vi "MainExpTrainCode.vi"() -> ()   [LabVIEW 2013]
uses:
  <vilib>/Utility/error.llb/DialogType.ctl
  <vilib>/DAQmx/write.llb/DAQmx Write (Analog Wfm 1Chan NSamp).vi
  <vilib>/DAQmx/create/channels.llb/DAQmx Create Channel (AO-Voltage-Basic).vi
  <vilib>/DAQmx/configure/timing.llb/DAQmx Timing (Sample Clock).vi
  <vilib>/DAQmx/miscellaneous.llb/DAQmx Fill In Error Info.vi
  <resource>/objmgr/daqmx.rc
  <vilib>/measure/NI_MAPro.lvlib
panel:
  in  "offset (volt)":dbl format="%0.2p"
  in  "Time Constant (us)":dbl=50.0
  in  "frequency (Hz)":dbl=10.0 format="%0.2p"
  in  "amplitude (volt)":dbl=1.0 format="%0.2p"
  in  "Number of Samples":i32=1000
  in  "Clock Source":tag="OnboardClock"
  out "Actual Sampling rate (S/s)":dbl=200000.0
  in  "Sample rate( S/s)":dbl=200000.0 format="%0.2f"
  out "Waveform Chart":waveform(dbl)(graph)={"t0"=timestamp(0 s since 1904-01-01), "dt"=5e-06, "Y"=array[1000 elements]}
  in  "stop":bool
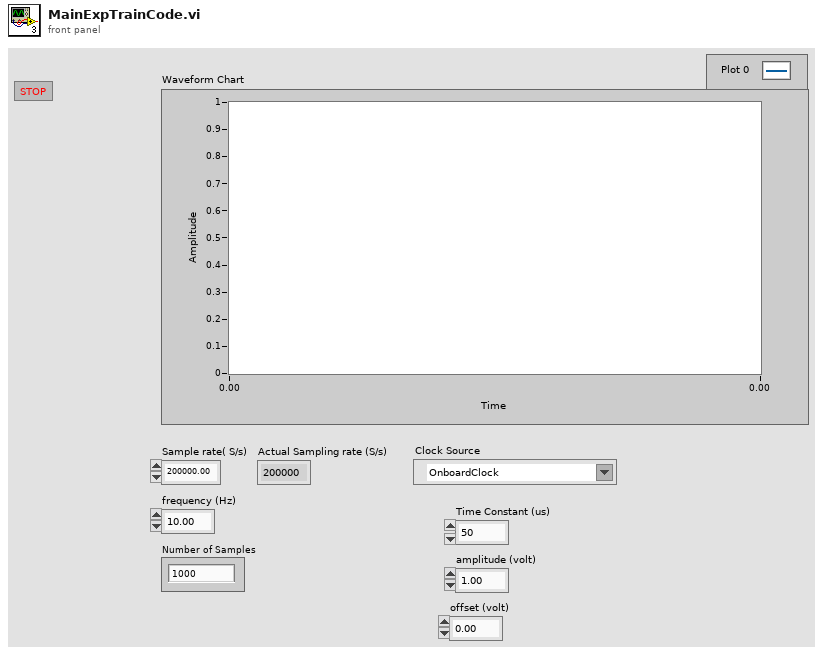
[diagram p1: front panel]
types:
  T1 = typedef "DialogType.ctl" = u16
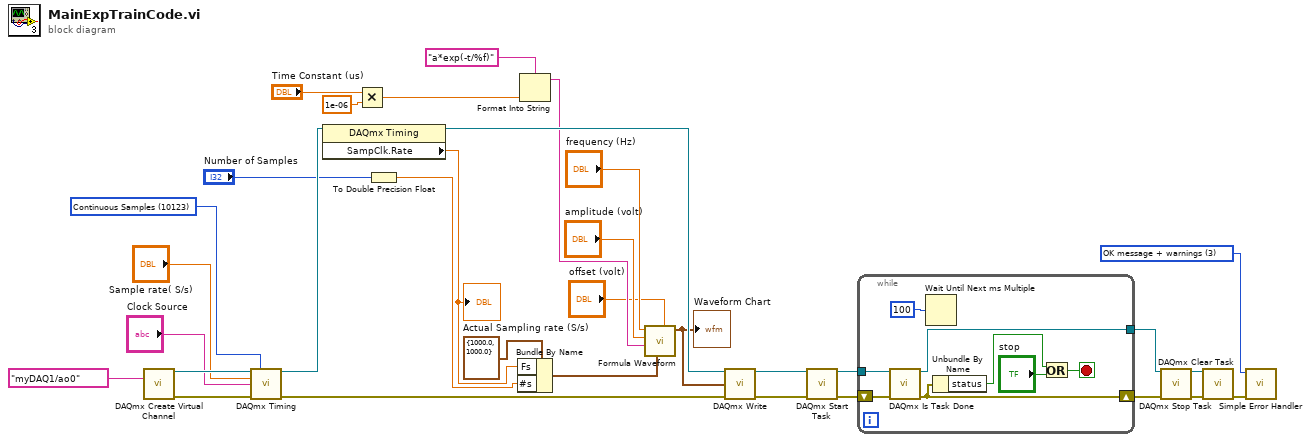
[diagram p0: block diagram]
diagram:
  w10 = T1 3 items=["no dialog", "OK message", "continue or stop message", "OK message + warnings", "continue/stop + warnings"] ("type of dialog (OK msg:1)")
  w32 = 10123 items=["Finite Samples"=10178, "Continuous Samples"=10123, "Hardware Timed Single Point"=12522] ("sample mode")
  n1 = call-poly <vilib>:"DAQmx Create Virtual Channel.vi"("physical channels"=tag "myDAQ1/ao0") -> ("task out"=w27:refnum<k21>, "error out"=w26:errorcluster)  [unwired: 13 in]
  n2 = call-poly <vilib>:"DAQmx Timing.vi"("task/channels in"=w27, "sample mode"=w32, "rate"="Sample rate( S/s)", "source"="Clock Source", "error in"=w26) -> ("task out"=w24:refnum<k21>, "error out"=w15:errorcluster)  [unwired: 9 in]
  n3 = property class="DAQmx Timing"(reference=w24) -> (reference out=w16:refnum<k21>, "SampClk.Rate"=w21:dbl)  [unwired: 1 in, 1 out]
  "Actual Sampling rate (S/s)" <- w21
  n4 = Multiply(x="Time Constant (us)", y=1e-06) -> (x*y=w2:dbl)
  n5 = To Double Precision Float(number="Number of Samples") -> (double precision float=w19:dbl)
  n6 = Bundle By Name(cluster=cluster{"Fs":dbl, "#s":dbl} {"Fs"=1000.0, "#s"=1000.0} ("sampling info"), "Fs"=w21, "#s"=w19) -> (w18:cluster{"Fs":dbl, "#s":dbl})
  n7 = Format Into String(format string="a*exp(-t/%f)" ("formula"), w2) -> (resulting string=w5:string)  [unwired: 2 in, 1 out]
  n8 = call <vilib>:"Formula Waveform.vi"("offset"="offset (volt)", "sampling info"=w18, "formula"=w5, "amplitude"="amplitude (volt)", "frequency"="frequency (Hz)") -> ("signal out"=w9:waveform(dbl))  [unwired: 5 in, 1 out]
  "Waveform Chart" <- w9
  n9 = call-poly <vilib>:"DAQmx Write.vi"("task/channels in"=w16, "data"=w9, "error in"=w15) -> ("task out"=w17:refnum<k21>, "error out"=w14:errorcluster)  [unwired: 10 in, 1 out]
  n10 = call <vilib>:"DAQmx Start Task.vi"("task/channels in"=w17, "error in"=w14) -> ("task out"=w31:refnum<k21>, "error out"=w30:errorcluster)  [unwired: 12 in]
  n11 = while {
    shift-right: [w34] -> w28
    shift-left: w30 -> [w35]
    tunnel: w31 -> [w37]
    tunnel: [w36] -> w29
    stop <- w38 stop-if-true
    n12 = call <vilib>:"DAQmx Is Task Done.vi"("task/channels in"=w37, "error in"=w35) -> ("task out"=w36:refnum<k21>, "error out"=w34:errorcluster)  [unwired: 11 in, 1 out]
    n13 = Wait Until Next ms Multiple(millisecond multiple=u32 100) -> ()  [unwired: 1 out]
    n14 = Unbundle By Name(w34) -> ("status"=w41:bool)
    n15 = Or(x=w41, y="stop") -> (x .or. y?=w38:bool)
  }
  n16 = call <vilib>:"DAQmx Stop Task.vi"("task/channels in"=w29, "error in"=w28) -> ("task out"=w13:refnum<k21>, "error out"=w12:errorcluster)  [unwired: 12 in]
  n17 = call <vilib>:"DAQmx Clear Task.vi"("task in"=w13, "error in"=w12) -> ("error out"=w11:errorcluster)  [unwired: 13 in]
  n18 = call <vilib>:"Simple Error Handler.vi"("error code (no error:0)"=w10, "error in (no error)"=w11) -> ()  [unwired: 3 in, 5 out]
